vi "Test Request from String.vi"() -> ()   [LabVIEW 2020]
uses:
  HTTP Utils/Method.ctl
  HTTP Utils/Request/Request.lvclass
  <vilib>/IlluminatedG/lv-stream/URI/URI.lvclass
  HTTP Utils/HTTP Utils.lvlib
panel:
  out "Parse Error":errorcluster
  out "Body":string
  out "Headers":cluster{"Header":string, "Value":string}[](array[cluster])=[{"Header"="accept-encoding", "Value"="gzip, deflate"}, {"Header"="accept-language", "Value"="en-us"}, {"Header"="connection", "Value"="Keep-Alive"}, {"Header"="host", "Value"="www.tutorialspoint.com"}, {"Header"="user-agent", "Value"="Mozilla/4.0 (compatible; MSIE5.01; Windows NT)"}]
  out "Version String":string="HTTP/1.1"
  out "Method":T1
  out "Target":string="/hello.htm"
  in  "Request String":string="GET /hello.htm HTTP/1.1\r\nUser-Agent: Mozilla/4.0 (compatible; MSIE5.01; Windows NT)\r\nHost: www.tutorialspoint.com\r\nAccept-Language: en-us\r\nAccept-Encoding: gzip, deflate\r\nConnection: Keep-Alive\r\n\r\n"
  # "Ensure that lines end with '\\r\\n' and not just '\\n' for proper operation. Additionally, there must be a blank line at the end to not generate an error; the string needs to end with '\\r\\n\\r\\n'."
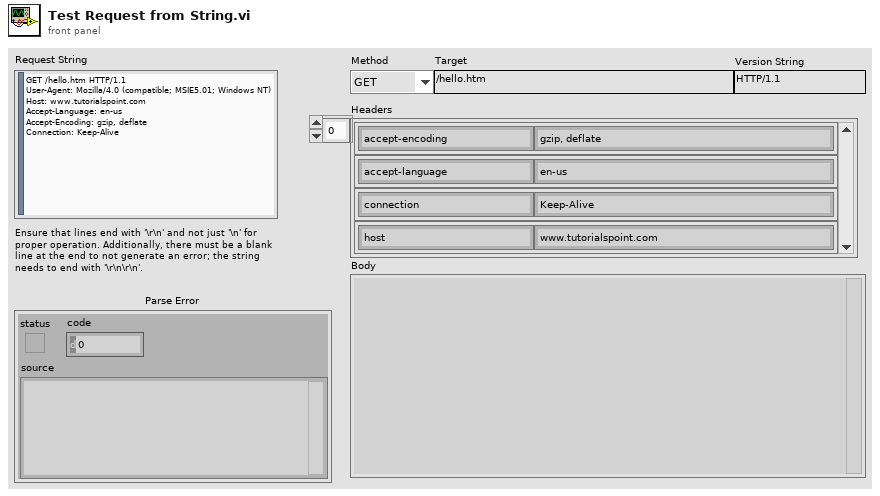
[diagram p1: front panel]
types:
  T1 = typedef "HTTP Utils.lvlib/Method.ctl" = enum16{"GET", "HEAD", "POST", "PUT", "DELETE", "CONNECT", "OPTIONS", "TRACE", "PATCH"}
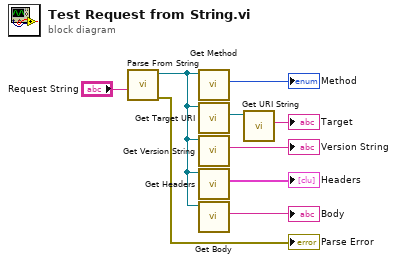
[diagram p0: block diagram]
diagram:
  n1 = call "Parse From String.vi"("Request String"="Request String") -> ("error out"=→"Parse Error":errorcluster, "Request out"=w8:refnum<class "Request.lvclass">)  [unwired: 9 in]
  n2 = call "Get Method.vi"("Request in"=w8) -> ("Method"=→"Method":T1)  [unwired: 8 in, 2 out]
  n3 = call "Get Target URI.vi"("Request in"=w8) -> ("Target URI"=w7:refnum<class "URI.lvclass">)  [unwired: 8 in, 2 out]
  n4 = call "Get Version String.vi"("Request in"=w8) -> ("Version String"=→"Version String":string)  [unwired: 8 in, 2 out]
  n5 = call "Get Headers.vi"("Request in"=w8) -> ("Headers"=→"Headers":cluster{"Header":string, "Value":string}[])  [unwired: 8 in, 2 out]
  n6 = call "Get Body.vi"("Request in"=w8) -> ("Body"=→"Body":string)  [unwired: 8 in, 2 out]
  n7 = call <vilib>:"Get URI String.vi"("URI in"=w7) -> ("URI String"=→"Target":string)  [unwired: 8 in, 2 out]
